vi "Copy Memory.vi"(8 "Error In":errorcluster, 9 "Copy Parameters":T1 {"Dimensions"."Width" min=1; "Dimensions"."Height" min=1; "Dimensions"."Depth" min=1}, 10 "Destination Object":T4 {"Dimension"."Width" min=1; "Dimension"."Height" min=1; "Dimension"."Depth" min=1}, 11 "Source Object":T4 {"Dimension"."Width" min=1; "Dimension"."Height" min=1; "Dimension"."Depth" min=1}) -> (0 "Error Out":errorcluster, 2 "Destination Object Out":T4 {"Dimension"."Width" min=1; "Dimension"."Height" min=1; "Dimension"."Depth" min=1}, 3 "Source Object Out":T4 {"Dimension"."Width" min=1; "Dimension"."Height" min=1; "Dimension"."Depth" min=1})   [LabVIEW 2012]
doc: "Copies a source memory object to a destination memory object.\n\nIf no copy parameters are given, OpenCLV checks if the arrays are the same size. If they are, the copy executes, otherwise an error is thrown."
uses:
  Non-User VIs/Controls/Memory Object.ctl
  Non-User VIs/Controls/Device ID.ctl
  Non-User VIs/Controls/Memory ID.ctl
  User Controls/Array Dimensions.ctl
  Non-User VIs/Controls/Memory Type.ctl
  User Controls/Copy Parameters.ctl
  User Controls/Offset.ctl
  Non-User VIs/Error Checking/Add Error Functional Global.vi
  OpenCLV x64.lvlib
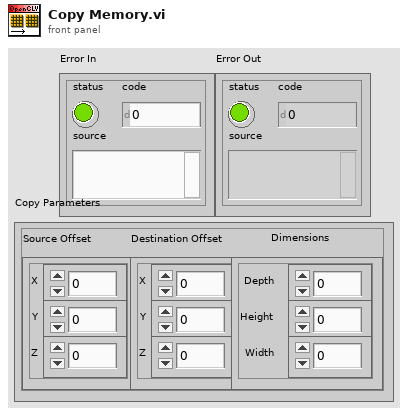
[diagram p1: front panel]
types:
  T1 = typedef "Copy Parameters.ctl" = cluster{"Source Offset":T2, "Destination Offset":T2, "Dimensions":T3}
  T2 = typedef "Offset.ctl" = cluster{"X":u64, "Y":u64, "Z":u64}
  T3 = typedef "Array Dimensions.ctl" = cluster{"Depth":u64, "Height":u64, "Width":u64}
  T4 = typedef "OpenCLV x64.lvlib/Memory Object.ctl" = cluster{"Device ID":T5, "Memeroy ID":T6, "Dimension":T3, "Memory Type":T7}
  T5 = typedef "OpenCLV x64.lvlib/Device ID.ctl" = u64
  T6 = typedef "OpenCLV x64.lvlib/Memory ID.ctl" = u64
  T7 = typedef "OpenCLV x64.lvlib/Memory Type.ctl" = enum16{"32f", "u8", "i8", "u16", "i16", "u32", "i32", "64f"}
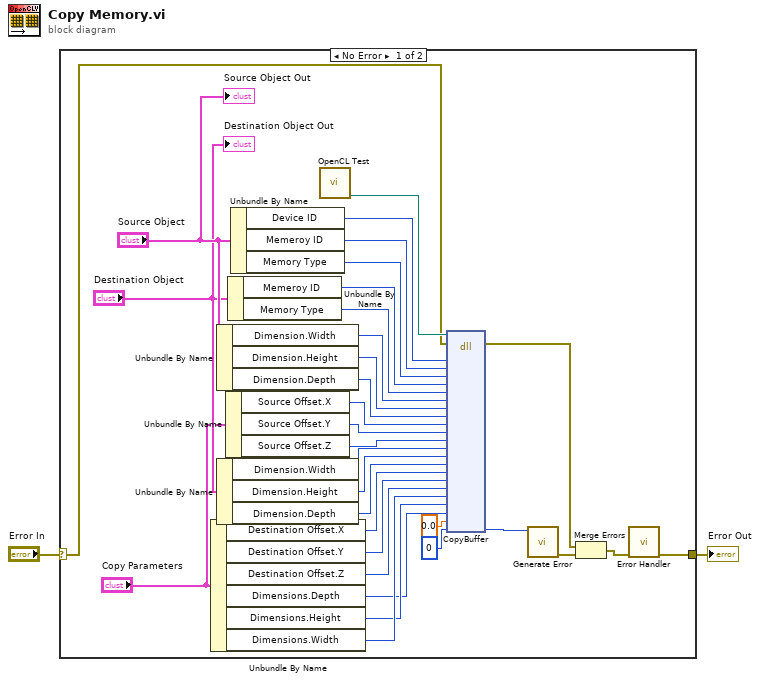
[diagram p0: block diagram]
diagram:
  n1 = case shown="No Error" "Error In" {
    selector: "Error In" -> [w6 w35]
    tunnel: [w34 w35] -> w1
    frame No Error {
      n2 = Unbundle By Name("Copy Parameters") -> ("Destination Offset.X"=w13:u64, "Destination Offset.Y"=w12:u64, "Destination Offset.Z"=w11:u64, "Dimensions.Depth"=w7:u64, "Dimensions.Height"=w8:u64, "Dimensions.Width"=w9:u64)
      n3 = Unbundle By Name("Source Object") -> ("Dimension.Width"=w23:u64, "Dimension.Height"=w22:u64, "Dimension.Depth"=w21:u64)
      n4 = Unbundle By Name("Destination Object") -> ("Dimension.Width"=w16:u64, "Dimension.Height"=w15:u64, "Dimension.Depth"=w14:u64)
      n5 = Unbundle By Name("Copy Parameters") -> ("Source Offset.X"=w20:u64, "Source Offset.Y"=w19:u64, "Source Offset.Z"=w18:u64)
      n6 = Unbundle By Name("Destination Object") -> ("Memeroy ID"=w26:T6, "Memory Type"=w25:T7)
      n7 = Unbundle By Name("Source Object") -> ("Device ID"=w29:T5, "Memeroy ID"=w28:T6, "Memory Type"=w27:T7)
      n8 = call "OpenCL Test.vi"() -> ("DLL To Use"=w31:path)  [unwired: 11 in]
      n9 = dll-call lib="C:/Users/bme-amcelroy-la/Desktop/OpenCLV/trunk/OpenCLV_x64_1.0/OpenCLV_x64.dll" fn="CopyBuffer"(path in=w31, error in=w6, "Labview Device"=w29, "Source Memory"=w28, "SourceType"=w27, "Dest"=w26, "DestType"=w25, "SrcWidth"=w23, "SrcHeight"=w22, "SrcDepth"=w21, "SrcXOffset"=w20, "SrcYOffset"=w19, "SrcZOffset"=w18, "DstWidth"=w16, "DstHeight"=w15, "DstDepth"=w14, "DstXOffset"=w13, "DstYOffset"=w12, "DstZOffset"=w11, "XRegion"=w9, "YRegion"=w8, "ZRegion"=w7, "Time"=0.0, "Error"=0) -> (error out=w3:errorcluster, "Error"=w33:i32)  [unwired: 23 in, 1 out]
      n10 = call "Generate Error.vi"("Error"=w33) -> ("error out"=w5:errorcluster)  [unwired: 10 in]
      n11 = Merge Errors(w3, w5) -> (w4:errorcluster)
      n12 = call-poly "Error Handler.vi"("Error In"=w4) -> ("Error Out"=w34:errorcluster)  [unwired: 10 in]
      "Destination Object Out" <- "Destination Object"
      "Source Object Out" <- "Source Object"
    }
    frame Error {
    }
  }
  "Error Out" <- w1
